vi "Anti-Spam Check.vi"(1 "No. of times the error has been handled in current One-Second Interval":u32) -> (0 "Need to handle this error?":bool)   [LabVIEW 2023, in "Error Manager.lvlib"]
doc: "The goal of the Anti-Spam Check is to prevent the Error Handler from having to handle* too many erros. \n\nWithout the Anti-Spam Check, the Error Handler can attempt to write too many errors to the log file, and to display too many errors in its GUI. This can lead to out-of-memory errors and the calling app hanging. This is obviously a serious user experience problem.\n\n*To handle = display in Error Handler GUI and log to file. 'handle' is a shorthand for multiple actions that the Error Handler performs when it needs to 'record' and error."
uses:
  Error Manager.lvlib
panel:
  out "Has the error already been handled enough times this second?":bool
  # "Development\nControls or indicators that are useful for development or testing, but which are not outputs of the VI."
  # "Input\nInputs to the VI"
  # "Output\nOutputs of the VI"
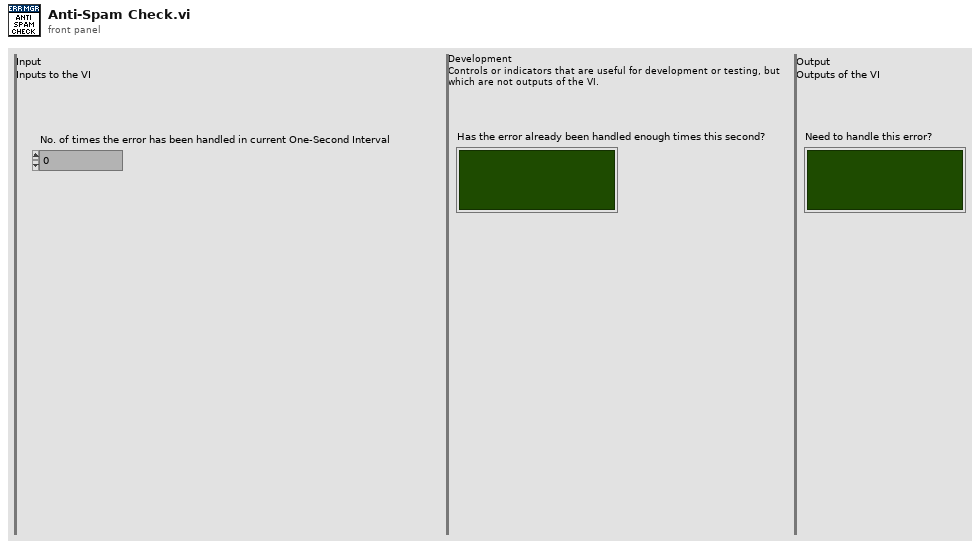
[diagram p1: front panel]
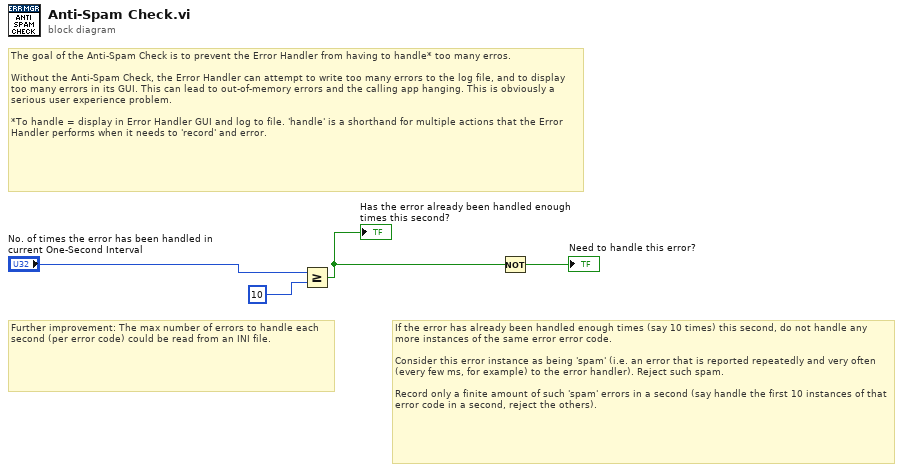
[diagram p0: block diagram]
diagram:
  # "If the error has already been handled enough times (say 10 times) this second, do not handle any more instances of the same error error code.\n\nConsider this error instance as being 'spam' (i.e. an error that is reported repeatedly and very often (every few ms, for example) to the error handler). Reject such spam. \n\nRecord only a finite amount of such 'spam' errors in a second (say handle the first 10 instances of that error code in a second, reject the others)."
  # "Further improvement: The max number of errors to handle each second (per error code) could be read from an INI file."
  # "The goal of the Anti-Spam Check is to prevent the Error Handler from having to handle* too many erros. \n\nWithout the Anti-Spam Check, the Error Handler can attempt to write too many errors to the log file, and to display too many errors in its GUI. This can lead to out-of-memory errors and the calling app hanging. This is obviously a serious user experience problem.\n\n*To handle = display in Error Handler GUI and log to file. 'handle' is a shorthand for multiple actions that the Error Handler performs when it needs to 'record' and error."
  n1 = Greater Or Equal?(x="No. of times the error has been handled in current One-Second Interval", y=u32 10) -> (x >= y?=w2:bool)
  "Has the error already been handled enough times this second?" <- w2
  n2 = Not(x=w2) -> (.not. x?=→"Need to handle this error?":bool)
